vi "快捷菜单激活(波形图表).vi"(11 "菜单引用":refnum<k9>) -> ()   [LabVIEW 2021]
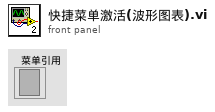
[diagram p1: front panel]
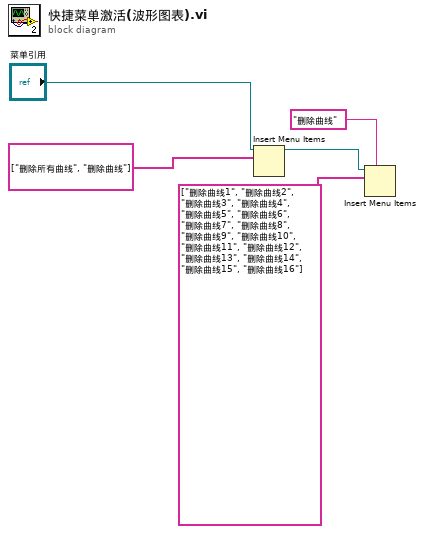
[diagram p0: block diagram]
diagram:
  n1 = Insert Menu Items ("插入菜单项")(8:string[] ["删除所有曲线", "删除曲线"] ("项名称"), 9:"菜单引用") -> (3:w3:refnum<k9>)  [unwired: 4 in, 2 out]
  n2 = Insert Menu Items ("插入菜单项")(5:"删除曲线" ("菜单标识符"), 8:string[] ["删除曲线1", "删除曲线2", "删除曲线3", "删除曲线4", "删除曲线5", "删除曲线6", "删除曲线7", "删除曲线8", "删除曲线9", "删除曲线10", "删除曲线11", "删除曲线12", "删除曲线13", "删除曲线14", "删除曲线15", "删除曲线16"] ("项名称"), 9:w3) -> ()  [unwired: 3 in, 3 out]
